vi "getRoot.vi"(8 "error in (no error)":errorcluster, 11 "LinkedList in":refnum<class "LinkedList.lvclass">) -> (0 "error out":errorcluster, 2 "Root":refnum<data-value>, 3 "LinkedList out":refnum<class "LinkedList.lvclass">)   [LabVIEW 2013, in "LinkedList.lvclass"]
doc: "Gets the root node (the frontmost node)."
uses:
  LinkedList.lvclass
  LLNode/LLNode.lvclass
  LinkedList.lvclass/LinkedList.ctl
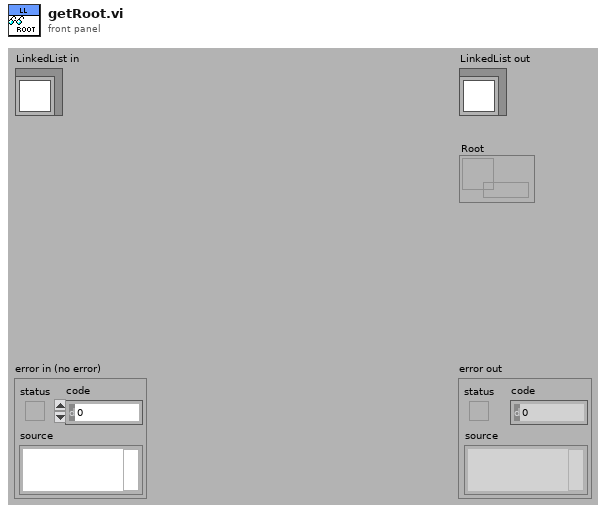
[diagram p1: front panel]
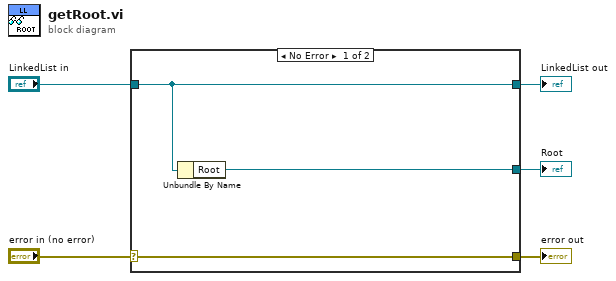
[diagram p0: block diagram]
diagram:
  n1 = case shown="No Error" "error in (no error)" {
    selector: "error in (no error)" -> [w8 w9]
    tunnel: [w8 w9] -> w4
    tunnel: [w7 w10] -> w2
    tunnel: "LinkedList in" -> [w7 w10]
    tunnel: [w6 _] -> w1
    frame No Error {
      n2 = Unbundle By Name(w7) -> ("Root"=w6:refnum<data-value>)
    }
    frame Error {
    }
  }
  "error out" <- w4
  "LinkedList out" <- w2
  "Root" <- w1
